vi "Control Climb.vi"   [LabVIEW 2020]
uses:
  Framework/Robot Global Data.vi
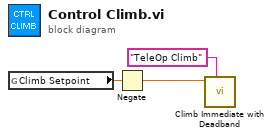
[diagram p0: block diagram]
diagram:
  n1 = global read "Robot Global Data.vi" "Climb Setpoint"() -> (w1:dbl)
  n2 = Negate(x=w1) -> (-x=w3:dbl)
  n3 = call "Climb Immediate with Deadband.vi"("Description"="TeleOp Climb", "Setpoint"=w3) -> ()  [unwired: 9 in, 1 out]
